vi "KGN beenden.vi"(8 "Fehler (Eingang, kein Fehler)":errorcluster, 11 "VISA-Ressourcenname":refnum<visa-resource-name>) -> (0 "Fehler (Ausgang)":errorcluster, 2 "Kommandos gesendet":string, 3 "VISA-Ressourcenname (Ausgang)":refnum<visa-resource-name>)   [LabVIEW 2020, in "Linearisierung v2.lvlib" / "Gasteiler.lvlib" / "HovaCAL_Interface.lvlib" / "KGN.lvlib"]
uses:
  KGN.lvlib
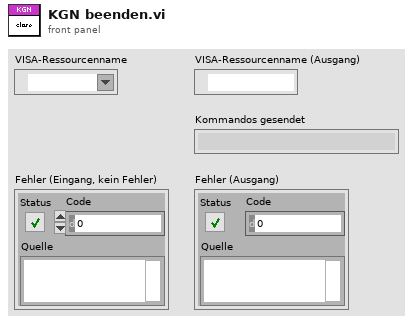
[diagram p1: front panel]
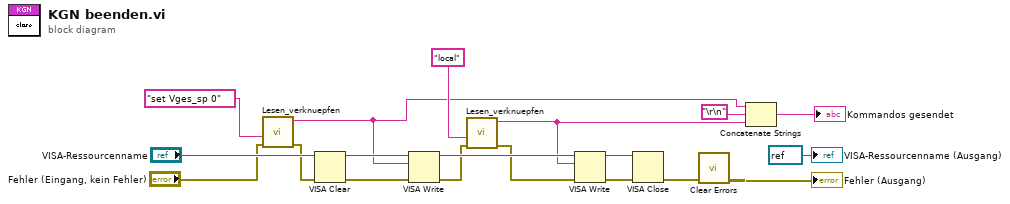
[diagram p0: block diagram]
diagram:
  n1 = call "Lesen_verknuepfen.vi"("error in (no error)"="Fehler (Eingang, kein Fehler)", "Order"="set Vges_sp 0" ("Schreibpuffer")) -> ("error out"=w5:errorcluster, "Verknüpfter String"=w1:string)  [unwired: 8 in]
  n2 = VISA Clear(VISA resource name="VISA-Ressourcenname", error in (no error)=w5) -> (VISA resource name out=w17:refnum<visa-resource-name>, error out=w14:errorcluster)
  n3 = VISA Write(VISA resource name=w17, write buffer=w1, error in (no error)=w14) -> (VISA resource name out=w19:refnum<visa-resource-name>, error out=w10:errorcluster)  [unwired: 1 out]
  n4 = call "Lesen_verknuepfen.vi"("error in (no error)"=w10, "Order"="local" ("Schreibpuffer")) -> ("error out"=w9:errorcluster, "Verknüpfter String"=w8:string)  [unwired: 8 in]
  n5 = VISA Write(VISA resource name=w19, write buffer=w8, error in (no error)=w9) -> (VISA resource name out=w16:refnum<visa-resource-name>, error out=w13:errorcluster)  [unwired: 1 out]
  n6 = VISA Close(VISA resource name=w16, error in (no error)=w13) -> (error out=w15:errorcluster)
  n7 = call <vilib>:"Clear Errors.vi"("error in (no error)"=w15) -> ("error out"=→"Fehler (Ausgang)":errorcluster)  [unwired: 5 in, 1 out]
  n8 = Concatenate Strings(w1, "\r\n", w8) -> (→"Kommandos gesendet":string)
  "VISA-Ressourcenname (Ausgang)" <- refnum<visa-resource-name> refnum ("VISA-Ressourcenname (Ausgang)")
